vi "ADIS16470 Loop.vi"(8 "error in":errorcluster) -> ()   [LabVIEW 2019]
uses:
  Typedef/ADIS16470 Device Reference.ctl
  Typedef/ADIS16470 Hardware Configuration.ctl
  <vilib>/Rock Robotics/WPI/SPI/WPI_SPIMode.ctl
  <vilib>/Rock Robotics/SystemInterfaces/DIO/FPGA_DIOChannel.ctl
  <vilib>/Rock Robotics/SystemInterfaces/spilib/spi_bus.ctl
  Typedef/ADIS16470 Status.ctl
  Typedef/ADIS16470 Data.ctl
  Typedef/ADIS16470 Process.ctl
  Typedef/ADIS16470 Command Type.ctl
  <vilib>/Rock Robotics/SystemInterfaces/CounterEncoderSourceConvertion/FPGA_CounterEncoderSourceConvertionLVSourceType.ctl
  <vilib>/Rock Robotics/SystemInterfaces/DIO/FPGA_DIODigitalSourceChannel.ctl
  <vilib>/Rock Robotics/SystemInterfaces/AnalogTrigger/FPGA_AnalogTriggerIndex.ctl
  <vilib>/Rock Robotics/SystemInterfaces/AnalogTrigger/FPGA_AnalogTriggerOutType.ctl
  Typedef/ADIS16470 Calibration Time.ctl
  <vilib>/Rock Robotics/WPI/SPI/WPI_SPIDevRef.ctl
  <vilib>/Rock Robotics/WPI/Interrupt/WPI_InterruptRef.ctl
  <vilib>/Rock Robotics/SystemInterfaces/Interrupt/FPGA_InterruptIndex.ctl
  Typedef/ADIS16470 Register.ctl
  <vilib>/Rock Robotics/WPI/Counter/WPI_CounterDigitalInputToDigitalSource.vi
panel:
  in  "Calibration Time":T1=enum."1s"
  in  "element":T2
  out "Waveform Chart":dbl(graph)
  out "Offset Bias":i16[](array[numeric])
  in  "ADIS16470DevRef":T3={"DevStatus"={"status"=FALSE, "code"=0, "source"=""}, "Hardware Config"={"SPI Clock Rate (Hz)"=1000000.0, "IMU SPI Mode (3)"=enum."Mode 3 (Clk Idle High,Sample on Trailing)", "IMU Reset Pin"=enum."SPI Port CS2", "IMU SPI Bus"=enum."SPI On-Board, CS0", "IMU Data Ready Pin"=enum."SPI Port CS1", "Stall Config"={"Pow2BytesPerRead"=255, "StallTicks"=640, "CsToSclkTicks"=5}}, "Calibration Complete"=refnum, "Status FIFO"=refnum, "Last Value Reference"=refnum, "Sychronous Process VI"=refnum, "Cmd FIFO"=refnum, "Source"={"DevStatus"={"status"=FALSE, "code"=0, "source"=""}, "AnalogTriggerMode?"=FALSE, "DigitalMode"={"DIO Channel"=enum."Disabled"}, "AnalogTriggerMode"={"AnalogTriggerIndex"=enum."Trig 0", "OutputType"=enum."InWindow"}}, "Data FIFO"=refnum, "Calibration Time"=enum."1s"}
  in  "Main Name":string
  # "XG_BIAS_LOW"
  # "XG_BIAS_HIGH"
  # "YG_BIAS_LOW"
  # "YG_BIAS_HIGH"
  # "ZG_BIAS_LOW"
  # "ZG_BIAS_HIGH"
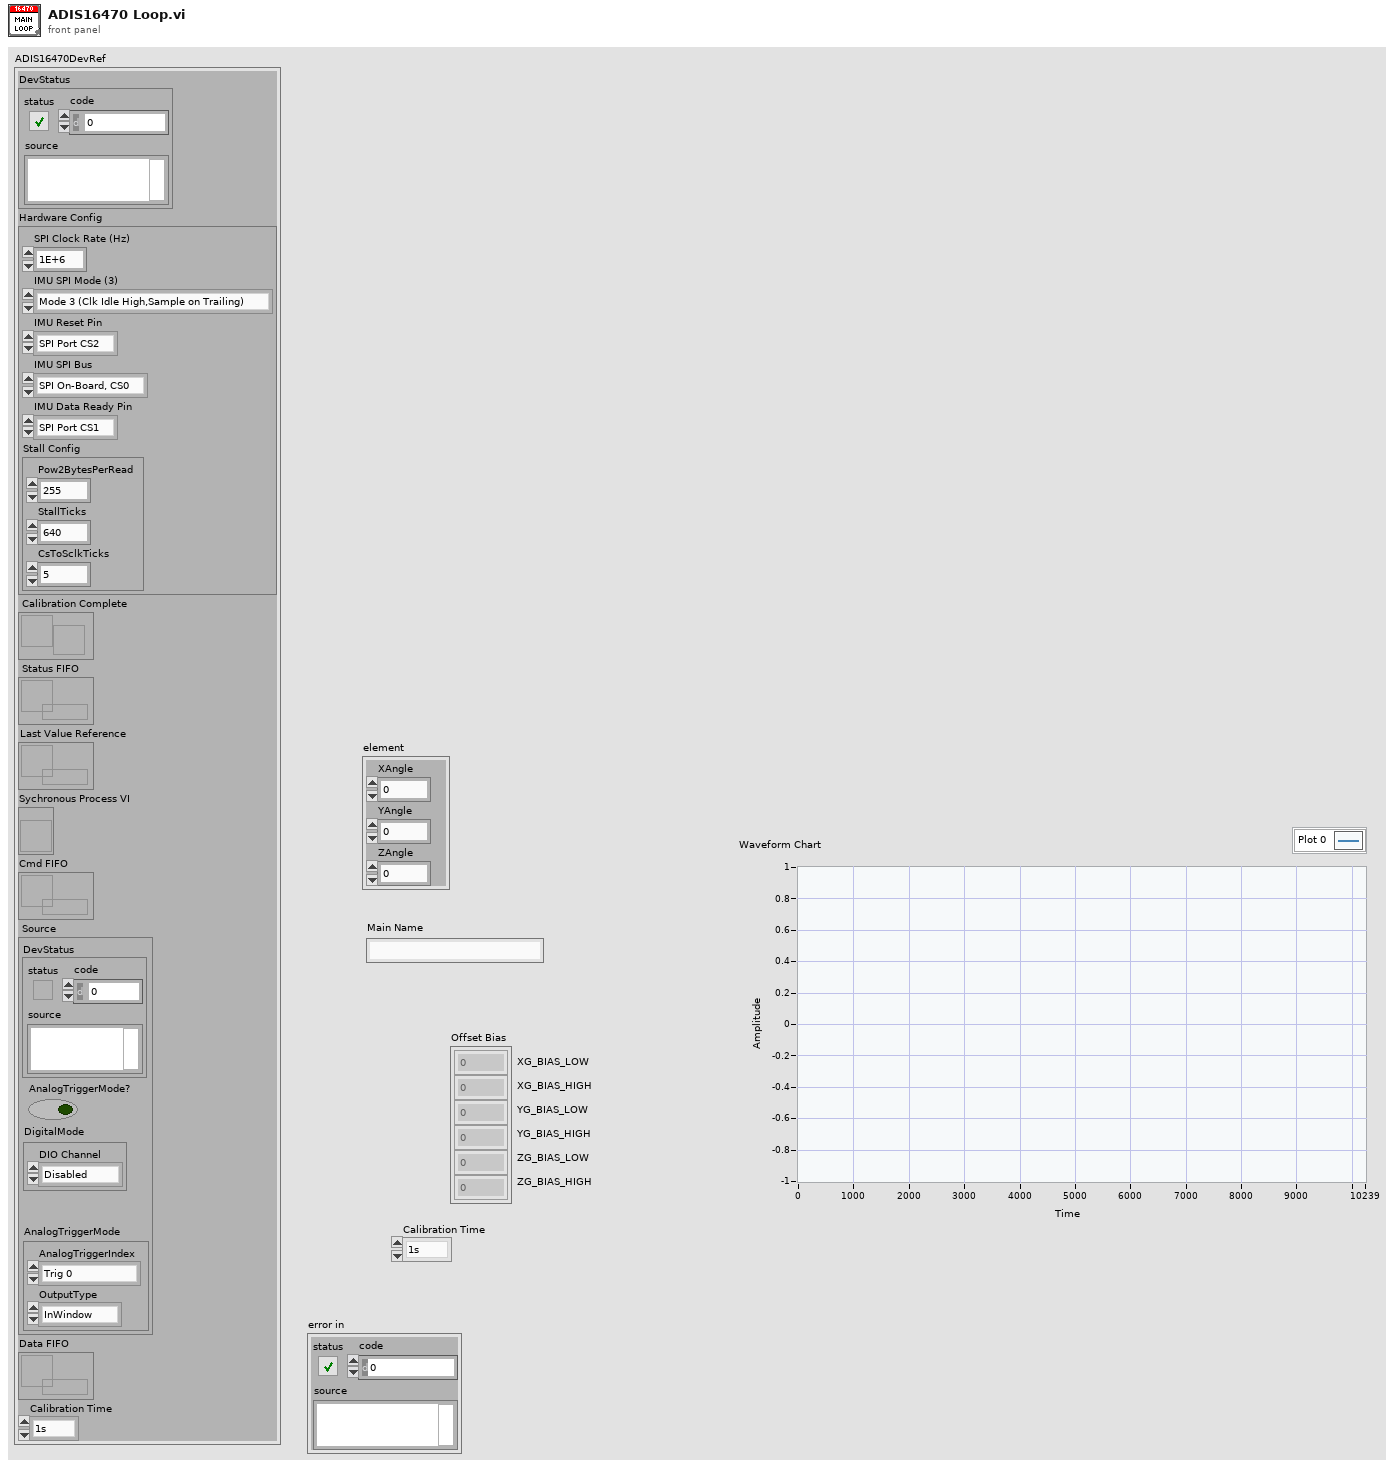
[diagram p1: front panel]
types:
  T1 = typedef "ADIS16470 Calibration Time.ctl" = enum16{"32ms", "64ms", "128ms", "256ms", "512ms", "1s", "2s", "4s", "8s", "16s", "32s", "64s"}
  T2 = typedef "ADIS16470 Data.ctl" = cluster{"XAngle":dbl, "YAngle":dbl, "ZAngle":dbl}
  T3 = typedef "ADIS16470 Device Reference.ctl" = cluster{"DevStatus":errorcluster, "Hardware Config":T4, "Calibration Complete":refnum<notifier>, "Status FIFO":refnum<k33>, "Last Value Reference":refnum<data-value>, "Sychronous Process VI":T8, "Cmd FIFO":refnum<k33>, "Source":T9, "Data FIFO":refnum<k33>, "Calibration Time":T1}
  T4 = typedef "ADIS16470 Hardware Configuration.ctl" = cluster{"SPI Clock Rate (Hz)":dbl, "IMU SPI Mode (3)":T5, "IMU Reset Pin":T6, "IMU SPI Bus":T7, "IMU Data Ready Pin":T6, "Stall Config":cluster{"Pow2BytesPerRead":u8, "StallTicks":u16, "CsToSclkTicks":u8}}
  T5 = typedef "WPI_SPIMode.ctl" = enum16{"Mode 0 (Clk Idle Low,Sample on Leading)", "Mode 1 (Clk Idle Low,Sample on Trailing)", "Mode 2 (Clk Idle High,Sample on Leading)", "Mode 3 (Clk Idle High,Sample on Trailing)"}
  T6 = typedef "FPGA_DIOChannel.ctl" = enum8{"DIO 0", "DIO 1", "DIO 2", "DIO 3", "DIO 4", "DIO 5", "DIO 6", "DIO 7", "DIO 8", "DIO 9", "DIO MXP 0", "DIO MXP 1", "DIO MXP 2", "DIO MXP 3", "DIO MXP 4", "DIO MXP 5", "DIO MXP 6", "DIO MXP 7", "DIO MXP 8", "DIO MXP 9", "DIO MXP 10", "DIO MXP 11", "DIO MXP 12", "DIO MXP 13", "DIO MXP 14", "DIO MXP 15", "SPI Port CS1", "SPI Port CS2", "SPI Port CS3", "SPI Port MISO", "SPI Port MOSI", "Invalid"}
  T7 = typedef "spi_bus.ctl" = enum16{"SPI On-Board, CS0", "SPI On-Board, CS1", "SPI On-Board, CS2", "SPI On-Board, CS3", "SPI MXP", "Invalid"}
  T8 = typedef "ADIS16470 Process.ctl" = refnum<vi>
  T9 = typedef "FPGA_CounterEncoderSourceConvertionLVSourceType.ctl" = cluster{"DevStatus":errorcluster, "AnalogTriggerMode?":bool, "DigitalMode":cluster{"DIO Channel":T10}, "AnalogTriggerMode":cluster{"AnalogTriggerIndex":T11, "OutputType":T12}}
  T10 = typedef "FPGA_DIODigitalSourceChannel.ctl" = enum8{"DIO 0", "DIO 1", "DIO 2", "DIO 3", "DIO 4", "DIO 5", "DIO 6", "DIO 7", "DIO 8", "DIO 9", "DIO MXP 0", "DIO MXP 1", "DIO MXP 2", "DIO MXP 3", "DIO MXP 4", "DIO MXP 5", "DIO MXP 6", "DIO MXP 7", "DIO MXP 8", "DIO MXP 9", "DIO MXP 10", "DIO MXP 11", "DIO MXP 12", "DIO MXP 13", "DIO MXP 14", "DIO MXP 15", "SPI Port CS1", "SPI Port CS2", "SPI Port CS3", "SPI Port MISO", "SPI Port MOSI", "Disabled"}
  T11 = typedef "FPGA_AnalogTriggerIndex.ctl" = enum8{"Trig 0", "Trig 1", "Trig 2", "Trig 3", "Trig 4", "Trig 5", "Trig 6", "Trig 7", "Invalid"}
  T12 = typedef "FPGA_AnalogTriggerOutType.ctl" = enum16{"InWindow", "TriggerState", "Rising", "Falling"}
  T13 = typedef "WPI_SPIDevRef.ctl" = cluster{"DevStatus":errorcluster, "Handle":i32, "SPI Bus":T7}
  T14 = typedef "WPI_InterruptRef.ctl" = cluster{"DevStatus":errorcluster, "InterruptIndex":T15}
  T15 = typedef "FPGA_InterruptIndex.ctl" = enum8{"0", "1", "2", "3", "4", "5", "6", "7", "Invalid"}
  T16 = cluster{"SPIDevRef":T13, "InterruptRef":T14, "Data Counter":u16, "Reset":bool, "Digital Source":T9, "Bytes Per Sample":u32, "Data":dbl[], "ADIS16470DevRef":T3, "TimeStampPrev":u32, "Sensor to Robot Rotation":dbl[][]}
  T17 = typedef "ADIS16470 Status.ctl" = cluster{"Calibrated?":bool}
  T18 = typedef "ADIS16470 Register.ctl" = u8
  T19 = typedef "ADIS16470 Command Type.ctl" = cluster{"Command":enum16{"None", "Reset", "Set Calibration Period", "Recalibrate", "Recal Complete"}, "Data":u32}
  T20 = typedef "WPI_DigitalOutputDevRef.ctl" = cluster{"DIO Channel":T6, "DevStatus":errorcluster}
  T21 = typedef "WPI_DigitalInputDevRef.ctl" = cluster{"DevStatus":errorcluster, "DIO Channel":T6}
  T22 = cluster{"Pow2BytesPerRead":u8, "StallTicks":u16, "CsToSclkTicks":u8}
  T23 = enum16{"None", "Reset", "Set Calibration Period", "Recalibrate", "Recal Complete"}
  T24 = enum32{"Bad", "Idle", "Run top level", "Running"}
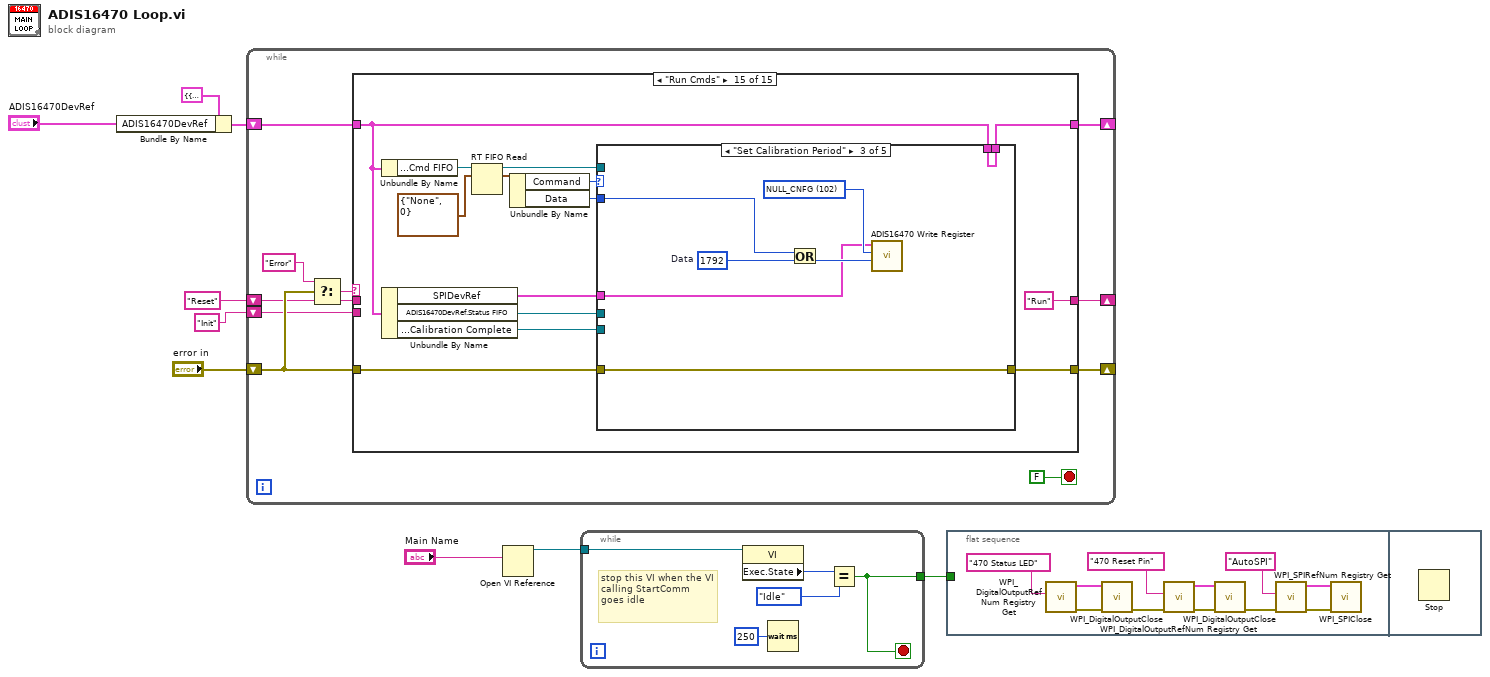
[diagram p0: block diagram]
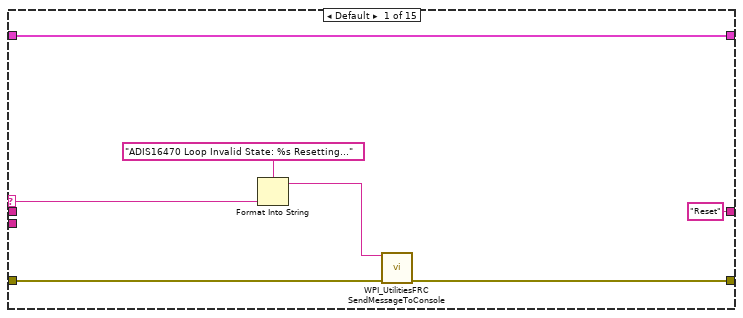
[diagram p2: hidden frame]
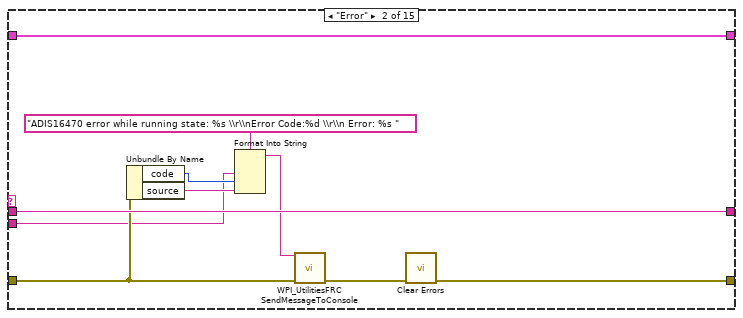
[diagram p3: hidden frame]
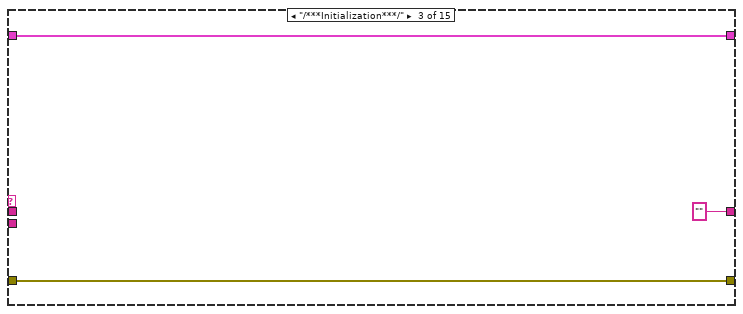
[diagram p4: hidden frame]
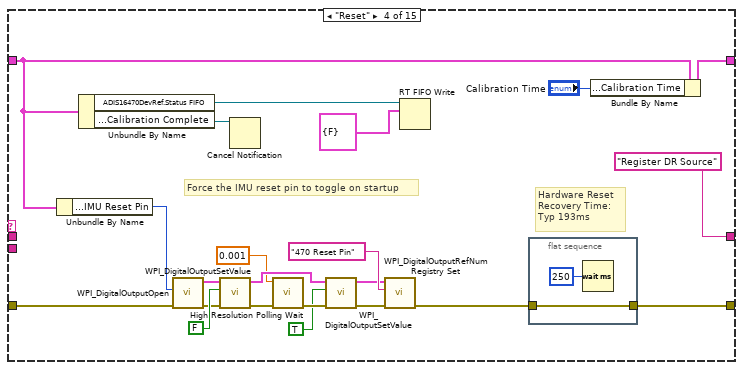
[diagram p5: hidden frame]
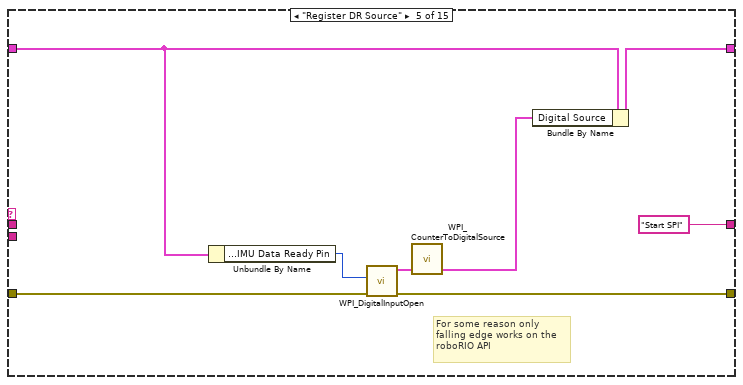
[diagram p6: hidden frame]
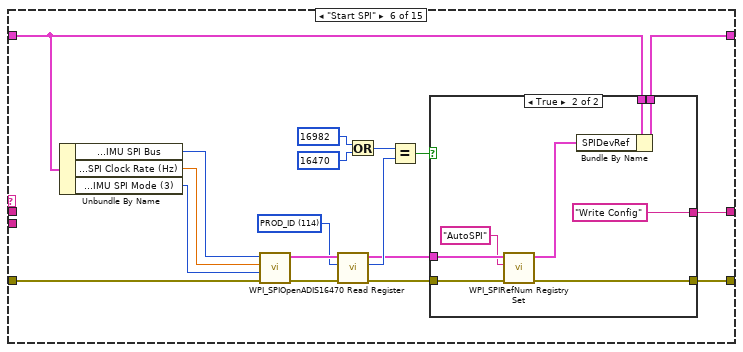
[diagram p7: hidden frame]
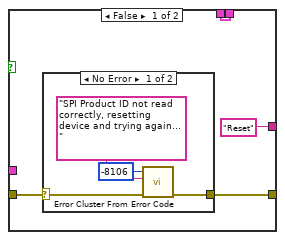
[diagram p8: hidden frame]
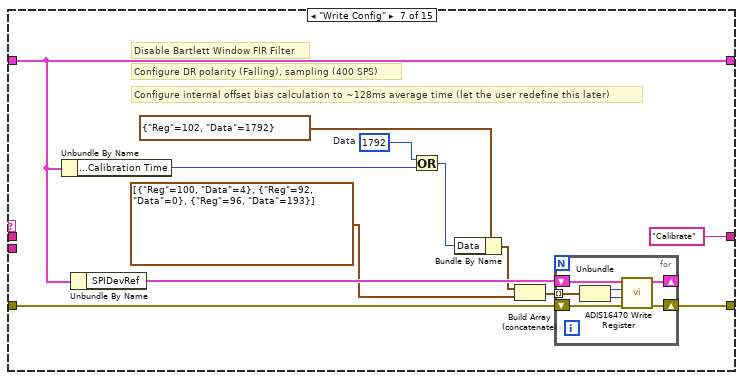
[diagram p10: hidden frame]
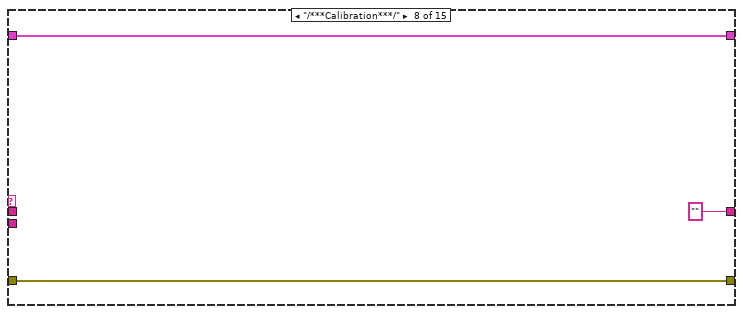
[diagram p11: hidden frame]
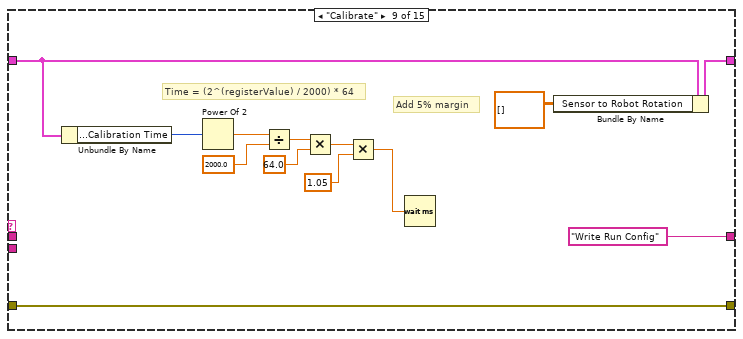
[diagram p12: hidden frame]
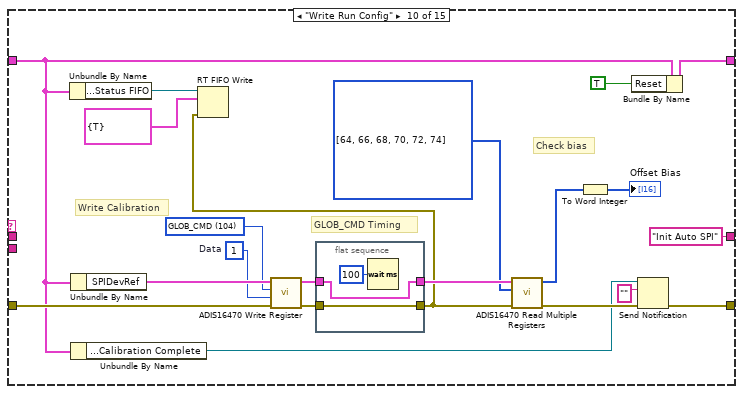
[diagram p13: hidden frame]
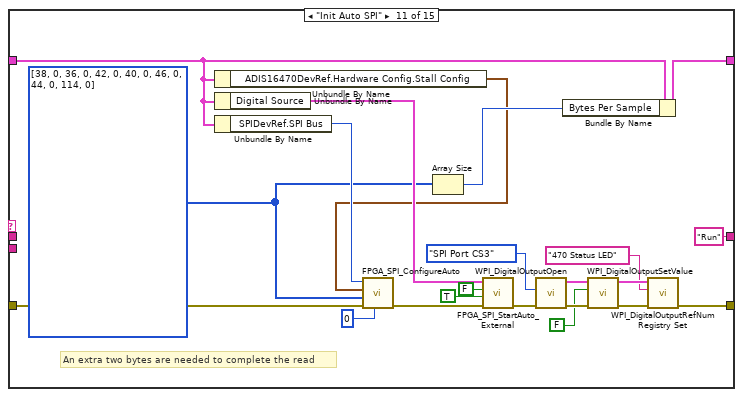
[diagram p14: hidden frame]
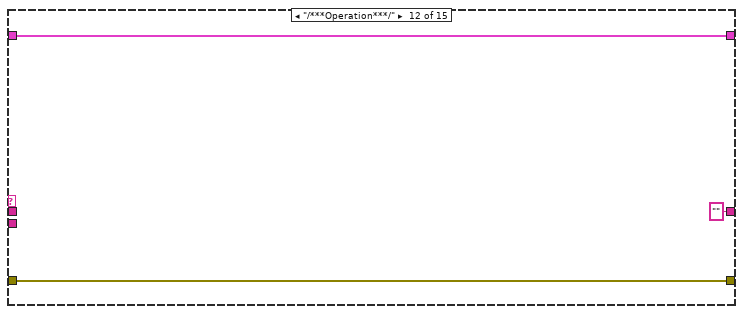
[diagram p15: hidden frame]
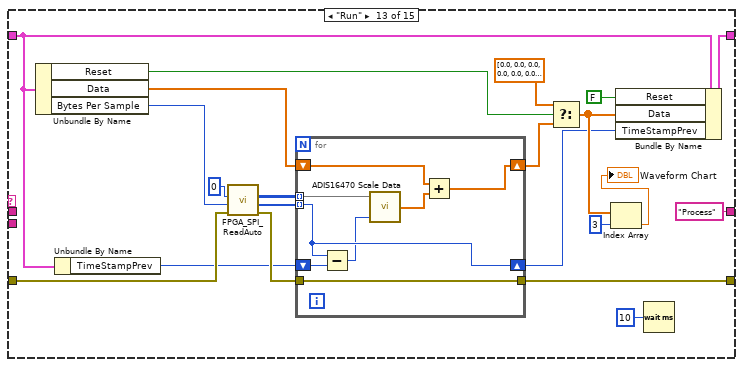
[diagram p16: hidden frame]
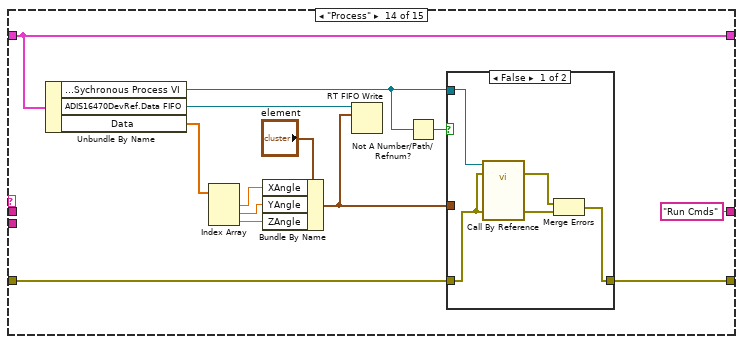
[diagram p17: hidden frame]
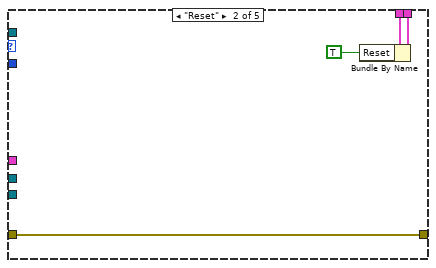
[diagram p20: hidden frame]
diagram:
  n1 = Bundle By Name(cluster=T16 {"SPIDevRef"={"DevStatus"={"status"=FALSE, "code"=0, "source"=""}, "Handle"=0, "SPI Bus"=enum."SPI On-Board, CS0"}, "InterruptRef"={"DevStatus"={"status"=FALSE, "code"=0, "source"=""}, "InterruptIndex"=enum."Invalid"}, "Data Counter"=0, "Reset"=FALSE, "Digital Source"={"DevStatus"={"status"=FALSE, "code"=0, "source"=""}, "AnalogTriggerMode?"=FALSE, "DigitalMode"={"DIO Channel"=enum."DIO 1"}, "AnalogTriggerMode"={"AnalogTriggerIndex"=enum."Trig 0", "OutputType"=enum."InWindow"}}, "Bytes Per Sample"=0, "Data"=[0.0, 0.0, 0.0, 0.0, 0.0, 0.0, 0.0, 0.0], "ADIS16470DevRef"={"DevStatus"={"status"=FALSE, "code"=0, "source"=""}, "Hardware Config"={"SPI Clock Rate (Hz)"=1000000.0, "IMU SPI Mode (3)"=enum."Mode 3 (Clk Idle High,Sample on Trailing)", "IMU Reset Pin"=enum."SPI Port CS2", "IMU SPI Bus"=enum."SPI On-Board, CS0", "IMU Data Ready Pin"=enum."SPI Port CS1", "Stall Config"={"Pow2BytesPerRead"=255, "StallTicks"=640, "CsToSclkTicks"=5}}, "Calibration Complete"=refnum, "Status FIFO"=refnum, "Last Value Reference"=refnum, "Sychronous Process VI"=refnum, "Cmd FIFO"=refnum, "Source"={"DevStatus"={"status"=FALSE, "code"=0, "source"=""}, "AnalogTriggerMode?"=FALSE, "DigitalMode"={"DIO Channel"=enum."Disabled"}, "AnalogTriggerMode"={"AnalogTriggerIndex"=enum."Trig 0", "OutputType"=enum."InWindow"}}, "Data FIFO"=refnum, "Calibration Time"=enum."1s"}, "TimeStampPrev"=0, "Sensor to Robot Rotation"=[]}, "ADIS16470DevRef"="ADIS16470DevRef") -> (w5:T16)
  n2 = while {
    shift-right: [w15] -> _
    shift-left: "Reset" -> [w12]
    shift-right: [w17] -> _
    shift-left: w5 -> [w18]
    shift-right: [w16] -> _
    shift-left: "error in" -> [w14]
    shift-left: "Init" -> [w10]
    stop <- FALSE stop-if-true
    n3 = Select(t="Error", s=w14, f=w12) -> (s? t:f=w13:string)
    n4 = case shown="\"Run Cmds\"" w13 {
      selector: w13 -> [w25 _ _ _ _ _ _ _ _ _ _ _ _ _ _]
      tunnel: w18 -> [w26 w36 w39 w42 w67 w79 w108 w128 w137 w146 w177 w190 w194 w231 w247]
      tunnel: [w26 w36 w39 w41 w70 w80 w108 w128 w140 w154 w176 w190 w210 w231 w248] -> w17
      tunnel: w14 -> [w24 w32 w38 w59 w69 w86 w116 w127 w139 w160 w186 w189 w207 w229 w250]
      tunnel: [w23 w33 w38 w57 w64 w78 w115 w127 w139 w148 w168 w189 w199 w228 w249] -> w16
      tunnel: ["Reset" w35 "" "Register DR Source" "Start SPI" w81 "Calibrate" "" "Write Run Config" "Init Auto SPI" "Run" "" "Process" "Run Cmds" "Run"] -> w15
      tunnel: w12 -> [_ w35 _ _ _ _ _ _ _ _ _ _ _ _ _]
      tunnel: w10 -> [_ w27 _ _ _ _ _ _ _ _ _ _ _ _ _]
      frame Default {
        n5 = Format Into String(format string="ADIS16470 Loop Invalid State: %s Resetting...", w25) -> (resulting string=w22:string)  [unwired: 2 in, 1 out]
        n6 = call <vilib>:"WPI_UtilitiesFRC SendMessageToConsole.vi"("Message"=w22, "error in (no error)"=w24) -> ("error out"=w23:errorcluster)  [unwired: 13 in]
      }
      frame "Error" {
        n7 = Unbundle By Name(w32) -> ("code"=w29:i32, "source"=w28:string)
        n8 = Format Into String(format string="ADIS16470 error while running state: %s \\r\\nError Code:%d \\r\\n Error: %s ", w27, w29, w28) -> (resulting string=w31:string)  [unwired: 2 in, 1 out]
        n9 = call <vilib>:"WPI_UtilitiesFRC SendMessageToConsole.vi"("Message"=w31, "error in (no error)"=w32) -> ("error out"=w34:errorcluster)  [unwired: 13 in]
        n10 = call <vilib>:"Clear Errors.vi"("error in (no error)"=w34) -> ("error out"=w33:errorcluster)  [unwired: 5 in, 1 out]
      }
      frame "/***Initialization***/" {
      }
      frame "Reset" {
        # "Hardware Reset Recovery Time: Typ 193ms"
        # "Force the IMU reset pin to toggle on startup"
        n11 = Unbundle By Name(w42) -> ("ADIS16470DevRef.Hardware Config.IMU Reset Pin"=w60:T6)
        n12 = Unbundle By Name(w42) -> ("ADIS16470DevRef.Status FIFO"=w55:refnum<k33>, "ADIS16470DevRef.Calibration Complete"=w56:refnum<notifier>)
        n13 = call <vilib>:"WPI_DigitalOutputOpen.vi"("error in (no error)"=w59, "DIO Channel"=w60) -> ("error out"=w52:errorcluster, "DigitalOutputDevRef"=w61:T20)  [unwired: 8 in]
        n14 = call <vilib>:"WPI_DigitalOutputSetValue.vi"("error in (no error)"=w52, "Value"=FALSE, "DigitalOutputDevRef"=w61) -> ("error out"=w49:errorcluster, "DigitalOutputDevRef"=w47:T20)  [unwired: 7 in]
        n15 = Cancel Notification(0:w56) -> ()  [unwired: 1 in, 3 out]
        n16 = call <vilib>:"High Resolution Polling Wait.vi"("error in (no error)"=w49, "seconds to wait"=0.001) -> ("error out"=w48:errorcluster)  [unwired: 9 in]
        n17 = call <vilib>:"WPI_DigitalOutputSetValue.vi"("error in (no error)"=w48, "Value"=TRUE, "DigitalOutputDevRef"=w47) -> ("error out"=w44:errorcluster, "DigitalOutputDevRef"=w45:T20)  [unwired: 7 in]
        n18 = call <vilib>:"WPI_DigitalOutputRefNum Registry Set.vi"("error in (no error)"=w44, "refnum name"="470 Reset Pin", "DigitalOutputDevRef"=w45) -> ("error out"=w50:errorcluster)  [unwired: 7 in, 1 out]
        n19 = RT FIFO Write(0:w55, 1:T17 {"Calibrated?"=FALSE} ("element")) -> ()  [unwired: 3 in, 4 out]
        n20 = flat-sequence {
          tunnel: [w63] -> w57
          tunnel: w50 -> [w63]
          frame #0 {
            n21 = Wait (ms)(milliseconds to wait=u32 250) -> ()  [unwired: 1 out]
          }
        }
        n22 = Bundle By Name(cluster=w42, "ADIS16470DevRef.Calibration Time"="Calibration Time") -> (w41:T16)
      }
      frame "Register DR Source" {
        # "For some reason only\nfalling edge works on the\nroboRIO API"
        n23 = Unbundle By Name(w67) -> ("ADIS16470DevRef.Hardware Config.IMU Data Ready Pin"=w66:T6)
        n24 = call <vilib>:"WPI_DigitalInputOpen.vi"("error in (no error)"=w69, "DIO Channel"=w66) -> ("error out"=w64:errorcluster, "DigitalInputDevRef"=w68:T21)  [unwired: 8 in]
        n25 = call-poly <vilib>:"WPI_CounterToDigitalSource.vi"("DigitalInputDevRef"=w68) -> ("Digital Source"=w65:T9)  [unwired: 6 in]
        n26 = Bundle By Name(cluster=w67, "Digital Source"=w65) -> (w70:T16)
      }
      frame "Start SPI" {
        w73 = T18 114 items=["Reserved1"=0, "DIAG_STAT"=2, "X_GYRO_LOW"=4, "X_GYRO_OUT"=6, "Y_GYRO_LOW"=8, "Y_GYRO_OUT"=10, "Z_GYRO_LOW"=12, "Z_GYRO_OUT"=14, "X_ACCL_LOW"=16, "X_ACCL_OUT"=18, "Y_ACCL_LOW"=20, "Y_ACCL_OUT"=22, "Z_ACCL_LOW"=24, "Z_ACCL_OUT"=26, "TEMP_OUT"=28, "TIME_STAMP"=30, "Reseved2"=32, "DATA_CNTR"=34, "X_DELTANG_LOW"=36, "X_DELTANG_OUT"=38, "Y_DELTANG_LOW"=40, "Y_DELTANG_OUT"=42, "Z_DELTANG_LOW"=44, "Z_DELTANG_OUT"=46, "X_DELTVEL_LOW"=48, "X_DELTVEL_OUT"=50, "Y_DELTVEL_LOW"=52, "Y_DELTVEL_OUT"=54, "Z_DELTVEL_LOW"=56, "Z_DELTVEL_OUT"=58, "Reserved3"=60, "Reserved4"=62, "XG_BIAS_LOW"=64, "XG_BIAS_HIGH"=66, "YG_BIAS_LOW"=68, "YG_BIAS_OUT"=70, "ZG_BIAS_LOW"=72, "ZG_BIAS_OUT"=74, "XA_BIAS_LOW"=76, "XA_BIAS_HIGH"=78, "YA_BIAS_LOW"=80, "YA_BIAS_OUT"=82, "ZA_BIAS_LOW"=84, "ZA_BIAS_OUT"=86, "Reserved5"=88, "Reserved6"=90, "FILT_CTRL"=92, "Reserved5"=94, "MSC_CTRL"=96, "UP_SCALE"=98, "DEC_RATE"=100, "NULL_CNFG"=102, "GLOB_CMD"=104, "Reserved6"=106, "FIRM_REV"=108, "FIRM_DM"=110, "FIRM_Y"=112, "PROD_ID"=114, "SERIAL_NUM"=116, "USER_SCR1"=118, "USER_SCR2"=120, "USER_SCR3"=122, "FLSHCNT_LOW"=124, "FLSHCNT_HIGH"=126] ("ADIS16448 Register")
        n27 = Unbundle By Name(w79) -> ("ADIS16470DevRef.Hardware Config.IMU SPI Bus"=w82:T7, "ADIS16470DevRef.Hardware Config.SPI Clock Rate (Hz)"=w83:dbl, "ADIS16470DevRef.Hardware Config.IMU SPI Mode (3)"=w84:T5)
        n28 = call <vilib>:"WPI_SPIOpen.vi"("error in"=w86, "Mode (3)"=w84, "Clock Rate (Hz)"=w83, "SPI Bus"=w82) -> ("error out"=w75:errorcluster, "SPIDevRef"=w74:T13)  [unwired: 6 in]
        n29 = call "ADIS16470 Read Register.vi"("error in (no error)"=w75, "ADIS16470 Register"=w73, "SPIDevRef in"=w74) -> ("error out"=w76:errorcluster, "Register Value"=w77:u16, "SPIDevRef out"=w72:T13)  [unwired: 6 in]
        n30 = Or(x=u16 16982 ("y"), y=u16 16470) -> (x .or. y?=w87:u16)
        n31 = Equal?(x=w87, y=w77) -> (x = y?=w85:bool)
        n32 = case shown="True" w85 {
          tunnel: ["Reset" "Write Config"] -> w81
          tunnel: w79 -> [w92 w105]
          tunnel: [w92 w104] -> w80
          tunnel: [w91 w100] -> w78
          tunnel: w76 -> [w90 w103]
          tunnel: w72 -> [_ w102]
          frame False {
            n33 = case shown="No Error" w90 {
              selector: w90 -> [w96 w98]
              tunnel: [w97 w98] -> w91
              frame No Error {
                n34 = call <vilib>:"Error Cluster From Error Code.vi"("error in (no error)"=w96, "error message (\"\")"="SPI Product ID not read correctly, resetting device and trying again..." ("error message (\"\")"), "error code (0)"=-8106) -> ("error out"=w97:errorcluster)  [unwired: 6 in]
              }
              frame Error {
              }
            }
          }
          frame True {
            n35 = call <vilib>:"WPI_SPIRefNum Registry Set.vi"("error in (no error)"=w103, "refnum name"="AutoSPI", "SPIDevRef"=w102) -> ("error out"=w100:errorcluster, "SPIDevRef"=w101:T13)  [unwired: 7 in]
            n36 = Bundle By Name(cluster=w105, "SPIDevRef"=w101) -> (w104:T16)
          }
        }
      }
      frame "Write Config" {
        w110 = 1792  # Data
        # "Configure internal offset bias calculation to ~128ms average time (let the user redefine this later)"
        # "Configure DR polarity (Falling), sampling (400 SPS)"
        # "Disable Bartlett Window FIR Filter"
        n37 = Unbundle By Name(w108) -> ("ADIS16470DevRef.Calibration Time"=w107:T1)
        n38 = Unbundle By Name(w108) -> ("SPIDevRef"=w117:T13)
        n39 = Or(x=w110, y=w107) -> (x .or. y?=w109:i32)
        n40 = Bundle By Name(cluster=cluster{"Reg":T18, "Data":i32} {"Reg"=102, "Data"=1792}, "Data"=w109) -> (w111:cluster{"Reg":T18, "Data":i32})
        n41 = Build Array (concatenate)(w111, cluster{"Reg":T18, "Data":u16}[] [{"Reg"=100, "Data"=4}, {"Reg"=92, "Data"=0}, {"Reg"=96, "Data"=193}]) -> (w112:cluster{"Reg":T18, "Data":i32}[])
        n42 = for {
          tunnel: w112 -> [w125] mode=indexing
          shift-right: [w121] -> w115
          shift-left: w116 -> [w120]
          shift-right: [w119] -> _
          shift-left: w117 -> [w122]
          n43 = Unbundle(w125) -> ("Reg"=w124:T18, "Data"=w123:i32)
          n44 = call "ADIS16470 Write Register.vi"("error in (no error)"=w120, "Data"=w123, "Register"=w124, "SPIDevRef in"=w122) -> ("error out"=w121:errorcluster, "SPIDevRef out"=w119:T13)  [unwired: 6 in]
        }
      }
      frame "/***Calibration***/" {
      }
      frame "Calibrate" {
        # "Add 5% margin"
        # "Time = (2^(registerValue) / 2000) * 64"
        n45 = Unbundle By Name(w137) -> ("ADIS16470DevRef.Calibration Time"=w136:T1)
        n46 = Power Of 2(x=w136) -> (2^x=w135:dbl)
        n47 = Divide(x=w135, y=2000.0) -> (x/y=w133:dbl)
        n48 = Multiply(x=w133, y=64.0) -> (x*y=w131:dbl)
        n49 = Multiply(x=w131, y=1.05) -> (x*y=w129:dbl)
        n50 = Wait (ms)(milliseconds to wait=w129) -> ()  [unwired: 1 out]
        n51 = Bundle By Name(cluster=w137, "Sensor to Robot Rotation"=dbl[][] []) -> (w140:T16)
      }
      frame "Write Run Config" {
        w143 = T18 104 items=["Reserved1"=0, "DIAG_STAT"=2, "X_GYRO_LOW"=4, "X_GYRO_OUT"=6, "Y_GYRO_LOW"=8, "Y_GYRO_OUT"=10, "Z_GYRO_LOW"=12, "Z_GYRO_OUT"=14, "X_ACCL_LOW"=16, "X_ACCL_OUT"=18, "Y_ACCL_LOW"=20, "Y_ACCL_OUT"=22, "Z_ACCL_LOW"=24, "Z_ACCL_OUT"=26, "TEMP_OUT"=28, "TIME_STAMP"=30, "Reseved2"=32, "DATA_CNTR"=34, "X_DELTANG_LOW"=36, "X_DELTANG_OUT"=38, "Y_DELTANG_LOW"=40, "Y_DELTANG_OUT"=42, "Z_DELTANG_LOW"=44, "Z_DELTANG_OUT"=46, "X_DELTVEL_LOW"=48, "X_DELTVEL_OUT"=50, "Y_DELTVEL_LOW"=52, "Y_DELTVEL_OUT"=54, "Z_DELTVEL_LOW"=56, "Z_DELTVEL_OUT"=58, "Reserved3"=60, "Reserved4"=62, "XG_BIAS_LOW"=64, "XG_BIAS_HIGH"=66, "YG_BIAS_LOW"=68, "YG_BIAS_OUT"=70, "ZG_BIAS_LOW"=72, "ZG_BIAS_OUT"=74, "XA_BIAS_LOW"=76, "XA_BIAS_HIGH"=78, "YA_BIAS_LOW"=80, "YA_BIAS_OUT"=82, "ZA_BIAS_LOW"=84, "ZA_BIAS_OUT"=86, "Reserved5"=88, "Reserved6"=90, "FILT_CTRL"=92, "Reserved5"=94, "MSC_CTRL"=96, "UP_SCALE"=98, "DEC_RATE"=100, "NULL_CNFG"=102, "GLOB_CMD"=104, "Reserved6"=106, "FIRM_REV"=108, "FIRM_DM"=110, "FIRM_Y"=112, "PROD_ID"=114, "SERIAL_NUM"=116, "USER_SCR1"=118, "USER_SCR2"=120, "USER_SCR3"=122, "FLSHCNT_LOW"=124, "FLSHCNT_HIGH"=126] ("Register")
        w159 = u16 1  # Data
        w155 = T18[] [64, 66, 68, 70, 72, 74] items=["Reserved1"=0, "DIAG_STAT"=2, "X_GYRO_LOW"=4, "X_GYRO_OUT"=6, "Y_GYRO_LOW"=8, "Y_GYRO_OUT"=10, "Z_GYRO_LOW"=12, "Z_GYRO_OUT"=14, "X_ACCL_LOW"=16, "X_ACCL_OUT"=18, "Y_ACCL_LOW"=20, "Y_ACCL_OUT"=22, "Z_ACCL_LOW"=24, "Z_ACCL_OUT"=26, "TEMP_OUT"=28, "TIME_STAMP"=30, "Reseved2"=32, "DATA_CNTR"=34, "X_DELTANG_LOW"=36, "X_DELTANG_OUT"=38, "Y_DELTANG_LOW"=40, "Y_DELTANG_OUT"=42, "Z_DELTANG_LOW"=44, "Z_DELTANG_OUT"=46, "X_DELTVEL_LOW"=48, "X_DELTVEL_OUT"=50, "Y_DELTVEL_LOW"=52, "Y_DELTVEL_OUT"=54, "Z_DELTVEL_LOW"=56, "Z_DELTVEL_OUT"=58, "Reserved3"=60, "Reserved4"=62, "XG_BIAS_LOW"=64, "XG_BIAS_HIGH"=66, "YG_BIAS_LOW"=68, "YG_BIAS_HIGH"=70, "ZG_BIAS_LOW"=72, "ZG_BIAS_HIGH"=74, "XA_BIAS_LOW"=76, "XA_BIAS_HIGH"=78, "YA_BIAS_LOW"=80, "YA_BIAS_HIGH"=82, "ZA_BIAS_LOW"=84, "ZA_BIAS_HIGH"=86, "Reserved5"=88, "Reserved6"=90, "FILT_CTRL"=92, "Reserved5"=94, "MSC_CTRL"=96, "UP_SCALE"=98, "DEC_RATE"=100, "NULL_CNFG"=102, "GLOB_CMD"=104, "Reserved6"=106, "FIRM_REV"=108, "FIRM_DM"=110, "FIRM_Y"=112, "PROD_ID"=114, "SERIAL_NUM"=116, "USER_SCR1"=118, "USER_SCR2"=120, "USER_SCR3"=122, "FLSHCNT_LOW"=124, "FLSHCNT_HIGH"=126] ("Registers")
        # "Write Calibration"
        # "GLOB_CMD Timing"
        # "Check bias"
        n52 = Unbundle By Name(w146) -> ("ADIS16470DevRef.Status FIFO"=w145:refnum<k33>)
        n53 = Unbundle By Name(w146) -> ("SPIDevRef"=w161:T13)
        n54 = Unbundle By Name(w146) -> ("ADIS16470DevRef.Calibration Complete"=w149:refnum<notifier>)
        n55 = RT FIFO Write(0:w145, 1:T17 {"Calibrated?"=TRUE} ("element"), 3:w142) -> ()  [unwired: 2 in, 4 out]
        n56 = call "ADIS16470 Write Register.vi"("error in (no error)"=w160, "Data"=w159, "Register"=w143, "SPIDevRef in"=w161) -> ("error out"=w158:errorcluster, "SPIDevRef out"=w157:T13)  [unwired: 6 in]
        n57 = flat-sequence {
          tunnel: w158 -> [w165]
          tunnel: [w165] -> w142
          tunnel: w157 -> [w163]
          tunnel: [w163] -> w156
          frame #0 {
            n58 = Wait (ms)(milliseconds to wait=u32 100) -> ()  [unwired: 1 out]
          }
        }
        n59 = call "ADIS16470 Read Multiple Registers.vi"("error in (no error)"=w142, "Registers"=w155, "SPIDevRef"=w156) -> ("error out"=w150:errorcluster, "Values"=w152:u16[])  [unwired: 7 in]
        n60 = To Word Integer(number=w152) -> (16bit integer=→"Offset Bias":i16[])
        n61 = Bundle By Name(cluster=w146, "Reset"=TRUE ("First Run")) -> (w154:T16)
        n62 = Send Notification(notification="", notifier=w149, error in (no error)=w150) -> (error out=w148:errorcluster)  [unwired: 1 out]
      }
      frame "Init Auto SPI" {
        w167 = T18[] [38, 0, 36, 0, 42, 0, 40, 0, 46, 0, 44, 0, 114, 0] items=["NULL"=0, "DIAG_STAT"=2, "X_GYRO_LOW"=4, "X_GYRO_OUT"=6, "Y_GYRO_LOW"=8, "Y_GYRO_OUT"=10, "Z_GYRO_LOW"=12, "Z_GYRO_OUT"=14, "X_ACCL_LOW"=16, "X_ACCL_OUT"=18, "Y_ACCL_LOW"=20, "Y_ACCL_OUT"=22, "Z_ACCL_LOW"=24, "Z_ACCL_OUT"=26, "TEMP_OUT"=28, "TIME_STAMP"=30, "Reseved2"=32, "DATA_CNTR"=34, "X_DELTANG_LOW"=36, "X_DELTANG_OUT"=38, "Y_DELTANG_LOW"=40, "Y_DELTANG_OUT"=42, "Z_DELTANG_LOW"=44, "Z_DELTANG_OUT"=46, "X_DELTVEL_LOW"=48, "X_DELTVEL_OUT"=50, "Y_DELTVEL_LOW"=52, "Y_DELTVEL_OUT"=54, "Z_DELTVEL_LOW"=56, "Z_DELTVEL_OUT"=58, "Reserved3"=60, "Reserved4"=62, "XG_BIAS_LOW"=64, "XG_BIAS_HIGH"=66, "YG_BIAS_LOW"=68, "YG_BIAS_HIGH"=70, "ZG_BIAS_LOW"=72, "ZG_BIAS_HIGH"=74, "XA_BIAS_LOW"=76, "XA_BIAS_HIGH"=78, "YA_BIAS_LOW"=80, "YA_BIAS_HIGH"=82, "ZA_BIAS_LOW"=84, "ZA_BIAS_HIGH"=86, "Reserved5"=88, "Reserved6"=90, "FILT_CTRL"=92, "Reserved5"=94, "MSC_CTRL"=96, "UP_SCALE"=98, "DEC_RATE"=100, "NULL_CNFG"=102, "GLOB_CMD"=104, "Reserved6"=106, "FIRM_REV"=108, "FIRM_DM"=110, "FIRM_Y"=112, "PROD_ID"=114, "SERIAL_NUM"=116, "USER_SCR1"=118, "USER_SCR2"=120, "USER_SCR3"=122, "FLSHCNT_LOW"=124, "FLSHCNT_HIGH"=126] ("Registers")
        # "An extra two bytes are needed to complete the read"
        n63 = Unbundle By Name(w177) -> ("ADIS16470DevRef.Hardware Config.Stall Config"=w166:T22)
        n64 = Unbundle By Name(w177) -> ("Digital Source"=w180:T9)
        n65 = Unbundle By Name(w177) -> ("SPIDevRef.SPI Bus"=w185:T7)
        n66 = call <vilib>:"FPGA_SPI_ConfigureAuto.vi"("SPI Auto Zero Byte Count"=u8 0, "error in"=w186, "SPI Auto TX Byte Array"=w167, "Stall Config"=w166, "SPI Bus"=w185) -> ("error out"=w183:errorcluster)  [unwired: 6 in]
        n67 = Array Size(array=w167) -> (size(s)=w175:i32)
        n68 = call <vilib>:"FPGA_SPI_StartAuto_External.vi"("error in (no error)"=w183, "Falling Edge"=TRUE, "Rising Edge"=FALSE, "Source"=w180) -> ("error out"=w178:errorcluster)  [unwired: 7 in]
        n69 = call <vilib>:"WPI_DigitalOutputOpen.vi"("error in (no error)"=w178, "DIO Channel"=FPGA_DIOChannel."SPI Port CS3") -> ("error out"=w174:errorcluster, "DigitalOutputDevRef"=w173:T20)  [unwired: 8 in]
        n70 = Bundle By Name(cluster=w177, "Bytes Per Sample"=w175) -> (w176:T16)
        n71 = call <vilib>:"WPI_DigitalOutputSetValue.vi"("error in (no error)"=w174, "Value"=FALSE, "DigitalOutputDevRef"=w173) -> ("error out"=w171:errorcluster, "DigitalOutputDevRef"=w170:T20)  [unwired: 7 in]
        n72 = call <vilib>:"WPI_DigitalOutputRefNum Registry Set.vi"("error in (no error)"=w171, "refnum name"="470 Status LED", "DigitalOutputDevRef"=w170) -> ("error out"=w168:errorcluster)  [unwired: 7 in, 1 out]
      }
      frame "/***Operation***/" {
      }
      frame "Run" {
        n73 = Unbundle By Name(w194) -> ("Reset"=w208:bool, "Data"=w202:dbl[], "Bytes Per Sample"=w206:u32)
        n74 = Unbundle By Name(w194) -> ("TimeStampPrev"=w193:u32)
        n75 = call <vilib>:"FPGA_SPI_ReadAuto.vi"("error in (no error)"=w207, "Bytes per Sample"=w206, "Samples to Read"=u32 0) -> ("error out"=w200:errorcluster, "Timestamps"=w203:u32[], "Data"=w204:u8[][])  [unwired: 6 in]
        n76 = for {
          tunnel: w204 -> [w213] mode=indexing
          tunnel: w203 -> [w216] mode=indexing
          shift-right: [w219] -> w201
          shift-left: w202 -> [w218]
          tunnel: w200 -> [w215]
          tunnel: [w215] -> w199
          shift-right: [w216] -> w192
          shift-left: w193 -> [w217]
          n77 = Subtract(x=w216, y=w217) -> (x-y=w212:u32)
          n78 = call "ADIS16470 Scale Data.vi"("TimeStamp"=w212, "Data In"=w213) -> ("Scaled Data Out"=w214:dbl[])  [unwired: 3 in]
          n79 = Add(x=w218, y=w214) -> (x+y=w219:dbl[])
        }
        n80 = Select(t=dbl[] [0.0, 0.0, 0.0, 0.0, 0.0, 0.0, 0.0, 0.0] ("Angle and Vel"), s=w208, f=w201) -> (s? t:f=w197:dbl[])
        n81 = Index Array(array=w197, index=3) -> (element=→"Waveform Chart":dbl)
        n82 = Bundle By Name(cluster=w194, "Reset"=FALSE ("First Run"), "Data"=w197, "TimeStampPrev"=w192) -> (w210:T16)
        n83 = Wait (ms)(milliseconds to wait=u32 10) -> ()  [unwired: 1 out]
      }
      frame "Process" {
        n84 = Unbundle By Name(w231) -> ("ADIS16470DevRef.Sychronous Process VI"=w226:T8, "ADIS16470DevRef.Data FIFO"=w230:refnum<k33>, "Data"=w225:dbl[])
        n85 = Index Array(array=w225) -> (element #1=w224:dbl, element #2=w223:dbl, element #3=w222:dbl)  [unwired: 3 in]
        n86 = Bundle By Name(cluster="element", "XAngle"=w224, "YAngle"=w223, "ZAngle"=w222) -> (w220:T2)
        n87 = RT FIFO Write(0:w230, 1:w220) -> ()  [unwired: 3 in, 4 out]
        n88 = Not A Number/Path/Refnum?(number/path/refnum=w226) -> (NaN/Path/Refnum?=w227:bool)
        n89 = case shown="False" w227 {
          tunnel: w229 -> [w233 w238]
          tunnel: w220 -> [_ _]
          tunnel: [w237 w238] -> w228
          tunnel: w226 -> [w236 _]
          frame False {
            n90 = call-by-ref "?"(reference=w236, error in=w233, 8:"error in (no error)"=w233) -> (error out=w234:errorcluster, 0:"error out"=w235:errorcluster)  [unwired: 10 in, 1 out]
            n91 = Merge Errors(w234, w235) -> (w237:errorcluster)
          }
          frame True {
          }
        }
      }
      frame "Run Cmds" {
        n92 = Unbundle By Name(w247) -> ("ADIS16470DevRef.Cmd FIFO"=w251:refnum<k33>)
        n93 = Unbundle By Name(w247) -> ("SPIDevRef"=w246:T13, "ADIS16470DevRef.Status FIFO"=w244:refnum<k33>, "ADIS16470DevRef.Calibration Complete"=w245:refnum<notifier>)
        n94 = RT FIFO Read(0:w251, 1:T19 {"Command"=enum."None", "Data"=0} ("element")) -> (8:w242:refnum<k33>, 9:w241:T19)  [unwired: 2 in, 3 out]
        n95 = Unbundle By Name(w241) -> ("Command"=w240:T23, "Data"=w239:u32)
        n96 = case shown="\"Set Calibration Period\"" w240 {
          tunnel: w247 -> [w253 w258 w265 w278 w287]
          tunnel: w250 -> [w254 w257 w264 w277 w286]
          tunnel: [w254 w257 w264 w277 w286] -> w249
          tunnel: [w253 w256 w265 w276 w287] -> w248
          tunnel: w246 -> [_ _ w259 w270 _]
          tunnel: w245 -> [_ _ _ _ w285]
          tunnel: w244 -> [_ _ _ w269 w283]
          tunnel: w242 -> [_ _ _ w267 _]
          tunnel: w239 -> [_ _ w260 _ _]
          frame "None", Default {
          }
          frame "Reset" {
            n97 = Bundle By Name(cluster=w258, "Reset"=TRUE ("First Run")) -> (w256:T16)
          }
          frame "Set Calibration Period" {
            w262 = T18 102 items=["Reserved1"=0, "DIAG_STAT"=2, "X_GYRO_LOW"=4, "X_GYRO_OUT"=6, "Y_GYRO_LOW"=8, "Y_GYRO_OUT"=10, "Z_GYRO_LOW"=12, "Z_GYRO_OUT"=14, "X_ACCL_LOW"=16, "X_ACCL_OUT"=18, "Y_ACCL_LOW"=20, "Y_ACCL_OUT"=22, "Z_ACCL_LOW"=24, "Z_ACCL_OUT"=26, "TEMP_OUT"=28, "TIME_STAMP"=30, "Reseved2"=32, "DATA_CNTR"=34, "X_DELTANG_LOW"=36, "X_DELTANG_OUT"=38, "Y_DELTANG_LOW"=40, "Y_DELTANG_OUT"=42, "Z_DELTANG_LOW"=44, "Z_DELTANG_OUT"=46, "X_DELTVEL_LOW"=48, "X_DELTVEL_OUT"=50, "Y_DELTVEL_LOW"=52, "Y_DELTVEL_OUT"=54, "Z_DELTVEL_LOW"=56, "Z_DELTVEL_OUT"=58, "Reserved3"=60, "Reserved4"=62, "XG_BIAS_LOW"=64, "XG_BIAS_HIGH"=66, "YG_BIAS_LOW"=68, "YG_BIAS_OUT"=70, "ZG_BIAS_LOW"=72, "ZG_BIAS_OUT"=74, "XA_BIAS_LOW"=76, "XA_BIAS_HIGH"=78, "YA_BIAS_LOW"=80, "YA_BIAS_OUT"=82, "ZA_BIAS_LOW"=84, "ZA_BIAS_OUT"=86, "Reserved5"=88, "Reserved6"=90, "FILT_CTRL"=92, "Reserved5"=94, "MSC_CTRL"=96, "UP_SCALE"=98, "DEC_RATE"=100, "NULL_CNFG"=102, "GLOB_CMD"=104, "Reserved6"=106, "FIRM_REV"=108, "FIRM_DM"=110, "FIRM_Y"=112, "PROD_ID"=114, "SERIAL_NUM"=116, "USER_SCR1"=118, "USER_SCR2"=120, "USER_SCR3"=122, "FLSHCNT_LOW"=124, "FLSHCNT_HIGH"=126] ("Register")
            w263 = 1792  # Data
            n98 = Or(x=w260, y=w263) -> (x .or. y?=w261:u32)
            n99 = call "ADIS16470 Write Register.vi"("Data"=w261, "Register"=w262, "SPIDevRef in"=w259) -> ()  [unwired: 7 in, 2 out]
          }
          frame "Recalibrate" {
            w271 = T18 104 items=["Reserved1"=0, "DIAG_STAT"=2, "X_GYRO_LOW"=4, "X_GYRO_OUT"=6, "Y_GYRO_LOW"=8, "Y_GYRO_OUT"=10, "Z_GYRO_LOW"=12, "Z_GYRO_OUT"=14, "X_ACCL_LOW"=16, "X_ACCL_OUT"=18, "Y_ACCL_LOW"=20, "Y_ACCL_OUT"=22, "Z_ACCL_LOW"=24, "Z_ACCL_OUT"=26, "TEMP_OUT"=28, "TIME_STAMP"=30, "Reseved2"=32, "DATA_CNTR"=34, "X_DELTANG_LOW"=36, "X_DELTANG_OUT"=38, "Y_DELTANG_LOW"=40, "Y_DELTANG_OUT"=42, "Z_DELTANG_LOW"=44, "Z_DELTANG_OUT"=46, "X_DELTVEL_LOW"=48, "X_DELTVEL_OUT"=50, "Y_DELTVEL_LOW"=52, "Y_DELTVEL_OUT"=54, "Z_DELTVEL_LOW"=56, "Z_DELTVEL_OUT"=58, "Reserved3"=60, "Reserved4"=62, "XG_BIAS_LOW"=64, "XG_BIAS_HIGH"=66, "YG_BIAS_LOW"=68, "YG_BIAS_OUT"=70, "ZG_BIAS_LOW"=72, "ZG_BIAS_OUT"=74, "XA_BIAS_LOW"=76, "XA_BIAS_HIGH"=78, "YA_BIAS_LOW"=80, "YA_BIAS_OUT"=82, "ZA_BIAS_LOW"=84, "ZA_BIAS_OUT"=86, "Reserved5"=88, "Reserved6"=90, "FILT_CTRL"=92, "Reserved5"=94, "MSC_CTRL"=96, "UP_SCALE"=98, "DEC_RATE"=100, "NULL_CNFG"=102, "GLOB_CMD"=104, "Reserved6"=106, "FIRM_REV"=108, "FIRM_DM"=110, "FIRM_Y"=112, "PROD_ID"=114, "SERIAL_NUM"=116, "USER_SCR1"=118, "USER_SCR2"=120, "USER_SCR3"=122, "FLSHCNT_LOW"=124, "FLSHCNT_HIGH"=126] ("Register")
            w274 = u16 1  # Data
            # "Write Calibration"
            # "GLOB_CMD Timing"
            n100 = RT FIFO Write(0:w269, 1:T17 {"Calibrated?"=FALSE} ("element")) -> ()  [unwired: 3 in, 4 out]
            n101 = call "ADIS16470 Write Register.vi"("Data"=w274, "Register"=w271, "SPIDevRef in"=w270) -> ("error out"=w273:errorcluster, "SPIDevRef out"=w272:T13)  [unwired: 7 in]
            n102 = RT FIFO Write(0:w267, 1:T19 {"Command"=enum."Recal Complete", "Data"=0} ("element")) -> ()  [unwired: 3 in, 4 out]
            n103 = flat-sequence {
              tunnel: w273 -> [w281]
              tunnel: [w281] -> _
              tunnel: w272 -> [w279]
              tunnel: [w279] -> _
              frame #0 {
                n104 = Wait (ms)(milliseconds to wait=u32 100) -> ()  [unwired: 1 out]
              }
            }
            n105 = Bundle By Name(cluster=w278, "Reset"=TRUE ("First Run")) -> (w276:T16)
          }
          frame "Recal Complete" {
            n106 = Send Notification(notification="", notifier=w285) -> ()  [unwired: 1 in, 2 out]
            n107 = RT FIFO Write(0:w283, 1:T17 {"Calibrated?"=TRUE} ("element")) -> ()  [unwired: 3 in, 4 out]
          }
        }
      }
    }
  }
  n108 = Open VI Reference(vi path="Main Name") -> (vi reference=w8:refnum<vi>)  [unwired: 3 in, 3 out]
  n109 = while {
    tunnel: w8 -> [w289]
    tunnel: [w288] -> w2
    stop <- w288 stop-if-true
    # "stop this VI when the VI calling StartComm goes idle"
    n110 = property class="VI"(reference=w289) -> ("Exec.State"=w291:T24)  [unwired: 1 in, 2 out]
    n111 = Wait (ms)(milliseconds to wait=u32 250) -> ()  [unwired: 1 out]
    n112 = Equal?(x=w291, y=T24."Idle" ("Execution:State")) -> (x = y?=w288:bool)
  }
  n113 = flat-sequence {
    tunnel: w2 -> [_]
    frame #0 {
      n114 = call <vilib>:"WPI_DigitalOutputRefNum Registry Get.vi"("refnum name"="470 Status LED") -> ("error out"=w302:errorcluster, "DigitalOutputDevRef"=w301:T20)  [unwired: 9 in]
      n115 = call <vilib>:"WPI_DigitalOutputClose.vi"("error in (no error)"=w302, "DigitalOutputDevRef"=w301) -> ("error out"=w300:errorcluster)  [unwired: 9 in]
      n116 = call <vilib>:"WPI_DigitalOutputRefNum Registry Get.vi"("error in (no error)"=w300, "refnum name"="470 Reset Pin") -> ("error out"=w298:errorcluster, "DigitalOutputDevRef"=w297:T20)  [unwired: 8 in]
      n117 = call <vilib>:"WPI_DigitalOutputClose.vi"("error in (no error)"=w298, "DigitalOutputDevRef"=w297) -> ("error out"=w296:errorcluster)  [unwired: 9 in]
      n118 = call <vilib>:"WPI_SPIRefNum Registry Get.vi"("error in (no error)"=w296, "refnum name"="AutoSPI") -> ("error out"=w294:errorcluster, "SPIDevRef"=w293:T13)  [unwired: 8 in]
      n119 = call <vilib>:"WPI_SPIClose.vi"("error in (no error)"=w294, "SPIDevRef"=w293) -> ()  [unwired: 9 in, 1 out]
    }
    frame #1 {
      n120 = Stop() -> ()  [unwired: 1 in]
    }
  }
